vi "Script_Excit_Check.vi"(8 "error in (no error)":errorcluster, 10 "Table of Waveforms":string[](array[string]), 11 "Number of excitations":i32=1 min=0 max=5 step=1) -> (0 "error out":errorcluster, 3 "Check Result":bool)   [LabVIEW 2018]
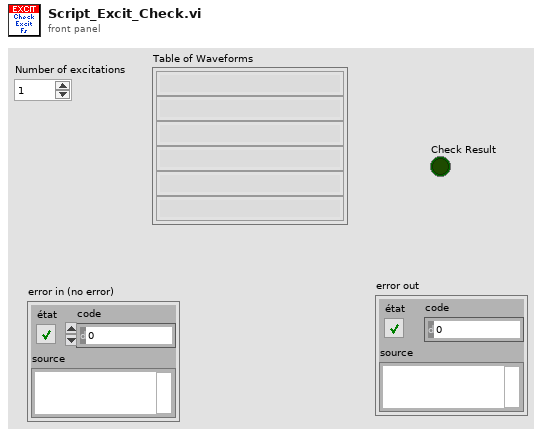
[diagram p1: front panel]
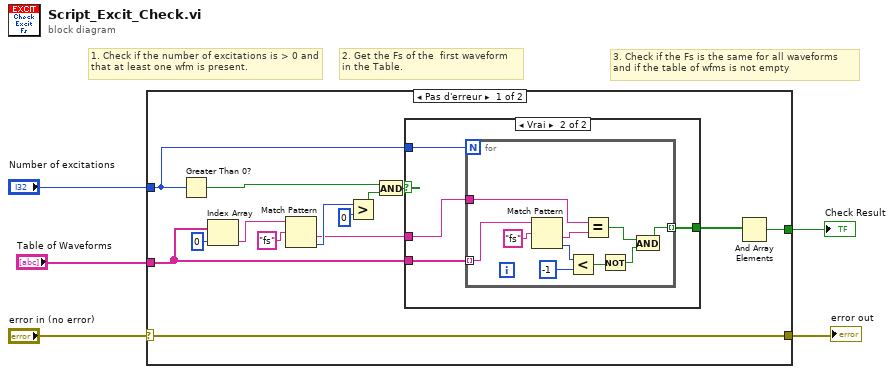
[diagram p0: block diagram]
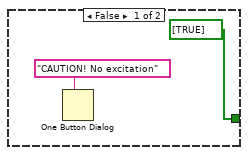
[diagram p2: hidden frame]
diagram:
  # "3. Check if the Fs is the same for all waveforms\nand if the table of wfms is not empty"
  # "2. Get the Fs of the  first waveform\nin the Table."
  # "1. Check if the number of excitations is > 0 and that at least one wfm is present."
  n1 = case shown="Pas d'erreur" "error in (no error)" {
    selector: "error in (no error)" -> [w18 w36]
    tunnel: [w18 w36] -> w4
    tunnel: "Table of Waveforms" -> [w11 _]
    tunnel: "Number of excitations" -> [w19 _]
    tunnel: [w16 _] -> w1
    frame No Error {
      n2 = Greater Than 0?(x=w19) -> (x > 0?=w15:bool)
      n3 = Index Array(array=w11, index=0 ("indice")) -> (element=w10:string)
      n4 = Match Pattern(string=w10, regular expression="fs" ("expression régulière")) -> (after substring=w6:string, offset past match=w9:i32)  [unwired: 1 in, 2 out]
      n5 = Greater?(x=w9, y=0) -> (0:w7:bool)
      n6 = And(x=w15, y=w7) -> (x .and. y?=w14:bool)
      n7 = case shown="Vrai" w14 {
        tunnel: w19 -> [_ w25]
        tunnel: w11 -> [_ w24]
        tunnel: [bool[] [TRUE] w23] -> w17
        tunnel: w6 -> [_ w22]
        frame False {
          n8 = One Button Dialog(message="CAUTION! No excitation") -> ()  [unwired: 1 in, 1 out]
        }
        frame True {
          n9 = for {
            N: w25 -> [_]
            tunnel: w24 -> [w35] mode=indexing
            tunnel: [w31] -> w23 mode=indexing
            tunnel: w22 -> [w26]
            n10 = Match Pattern(string=w35, regular expression="fs" ("expression régulière")) -> (after substring=w33:string, offset past match=w30:i32)  [unwired: 1 in, 2 out]
            n11 = Less?(x=w30, y=-1) -> (x < y?=w28:bool)
            n12 = Equal?(x=w26, y=w33) -> (x = y?=w32:bool)
            n13 = Not(x=w28) -> (.not. x?=w27:bool)
            n14 = And(x=w32, y=w27) -> (x .and. y?=w31:bool)
          }
        }
      }
      n15 = And Array Elements(Boolean array=w17) -> (logical AND=w16:bool)
    }
    frame Error {
    }
  }
  "error out" <- w4
  "Check Result" <- w1
